vi "Calibrate xtal.vi"(5 "External Attenuation, dB":T8 format="%.2f", 7 "CART TCP Connection In":refnum<k5>, 8 "Error In":errorcluster, 9 "Max Input Power, dBm":T7 format="%.1f", 11 "RFSA Device":T16="RFSA") -> (0 "error out":errorcluster)   [LabVIEW 2011]
doc: "(c) Copyright 2006, National Instruments, Inc. This VI may not be duplicated, sold, or distributed without written consent from National Instruments."
uses:
  <userlib>/niRF/niSystem/SA/Includes/niSYS - RFSA - INC - STYP - Handle.ctl
  <userlib>/niRF/niSystem/SA/Includes/niSYS - SA - INC - STYP - Trigger.ctl
  <userlib>/niRF/niSystem/SA/Includes/niSYS - SA - INC - STYP - Trigger Delay.ctl
  <userlib>/niRF/niSystem/SA/Includes/niSYS - SA - INC - STYP - Timeout.ctl
  <userlib>/niRF/niBasic/SA/Spectrum/Includes/niBASIC - SA - Spectrum - INC - STYP - Averaging.ctl
  <userlib>/niRF/niBasic/SA/Spectrum/Includes/niBASIC - SA - Spectrum - INC - STYP - Measurement.ctl
  <userlib>/niRF/niSystem/SA/Includes/niSYS - SA - INC - STYP - Frequency Reference.ctl
  <userlib>/niRF/niSystem/SA/Includes/niSYS - SA - INC - STYP - External Attenuation.ctl
  <userlib>/niRF/niSystem/SA/Includes/niSYS - SA - INC - STYP - Max Input Power.ctl
  <userlib>/niRF/niSystem/SA/Includes/niSYS - SA - INC - STYP - Center Frequency.ctl
  <userlib>/niRF/niBasic/SA/Spectrum/Includes/niBASIC - SA - Spectrum - INC - STYP - FFT Window.ctl
  <userlib>/niRF/niBasic/SA/Spectrum/Includes/niBASIC - SA - Spectrum - INC - STYP - Measurement RBW.ctl
  <userlib>/niRF/niSystem/SA/Includes/niSYS - SA - INC - STYP - Span.ctl
  <userlib>/niRF/niBasic/SA/Spectrum/Includes/niBASIC - SA - Spectrum - INC - STYP - FFT Size.ctl
  <userlib>/niRF/niBasic/SA/Spectrum/Includes/niBASIC - SA - Spectrum - INC - STYP - Filter Type.ctl
  WLAN/UUT/QCA/Controls/QCA NART Response Type.ctl
  <userlib>/niRF/niBasic/SA/Spectrum/Includes/niBASIC - SA - Spectrum - INC - STYP - Measurement Trace Type.ctl
  <userlib>/niRF/niSystem/SA/Includes/niSYS - SA - INC - STYP - Measurement Request.ctl
panel:
  in  "Filter Type":T1
  in  "FFT Size":T2={"Auto"=enum."On", "Min Pnts/RBW"=3.1, "Window Length"=706, "FFT Length"=1024} {"Min Pnts/RBW" format="%.1f"}
  in  "Span, Hz":T3=1000000.0 format="%^.3e"
  in  "Measurement RBW, Hz":T4={"Auto"=enum."On", "RBW, Hz"=1000000.0} {"RBW, Hz" format="%^.3e"}
  in  "FFT Window":T5
  in  "RFSA Center Frequency, Hz":T6=2437000000.0 format="%^.6e"
  out "Spectrum Graph":T9(graph)={999501953.125, "Time Domain Interval, sec"=4882.8125, "Waveform Measurement Trace"=[-94.58885960127041, -96.86839023376476, -99.44994709212702, -95.73980201325817, -94.85468685558206, -93.89939819937095, -92.96907780368053, -94.62427677362473, -96.00114334271848, -95.0773520951145, -94.62079733063136, -95.66039665905808, -97.26831199401815, -94.4245843897965, -94.11636842862069, -93.58322383773326, -96.15404542236388, -96.24945397470107, -95.50507217914763, -96.54108841377801, -96.20009898290628, -94.5853296471187, -92.45746866418841, -91.28538347271048, -91.87185526400654, -94.56638317616594, -96.80701098668649, -98.3947929158942, -98.51183674015738, -97.19248581591714, -96.81596744977271, -95.42900485531823, -95.06526491233971, -94.58696887517611, -95.97070348701587, -96.12508871585825, -96.44070407370447, -95.79000716907146, -97.40271981045801, -96.56026806674593, -96.63105214105727, -95.37951512730523, -95.0709837906345, -97.57170348129546, -98.65428166191879, -92.85960027957853, -90.69744081914348, -91.78092902523147, -93.01528314210488, -94.00436029202501, -93.35100459361215, -93.65439480062977, -94.03853395069989, -94.46526514886557, -94.89042305851434, -94.67424970039717, -93.63794705250254, -92.45925730447641, -92.65908155014344, -93.60044471338867, -94.45278046002886, -94.14161306416081, -95.1968357622903, -94.78018101642988, -94.3521734655379, -93.66111421566106, -94.84863517357037, -94.5954023919716, -96.31573035476218, -96.10673186698642, -95.71535800929679, -94.23828099215436, -93.52563000159624, -95.57033866863337, -95.53015116793134, -93.56809331780974, -92.7606452725199, -93.57072573308072, -95.32780281550693, -92.86665354898099, -93.1370950166728, -94.12900193004297, -94.87833817452723, -94.72912032302605, -94.17479444496155, -94.72686892886344, -93.6596877329905, -92.66964149507194, -93.08938347771124, -94.20661112927449, -97.92818192608922, -94.73725815144995, -93.72795972831032, -95.83148845299667, -93.96304770180853, -93.50544784378508, -92.44166060977277, -93.27927003206689, -87.23502888503836, -72.11564523212036, -65.2815070033974, -63.751961771120435, -63.76202638288482, -64.94683436227825, -71.0137879230945, -85.10120059441533, -91.83446895184292, -90.61921828145796, -90.72235231920887, -91.03886336724534, -91.42747554368565, -91.50468859500515, -90.91036635524621, -91.23961076459484, -93.16256151029376, -95.66587614800164, -96.70895620214242, -94.44704301225457, -93.34996435212136, -92.18571998503167, -92.8876926563818, -93.5060742547249, -94.69941271506612, -97.92708620913864, -95.25428896670476, -92.62306680566677, -91.3874988202419, -91.85885903026352, -93.43215873965788, -94.90985702146794, -94.99607107512729, -94.53014477422813, -94.84999122998677, -95.93647533060847, -95.05672593509198, -97.64855424631322, -95.46215659926096, -94.67802340702697, -94.36305677166051, -95.093191185747, -95.15591730271399, -94.6393427453004, -95.01042716486224, -93.48932052409448, -93.1088259750116, -95.79379158863588, -94.27401403528606, -94.39185567902642, -95.78566610842289, -96.2278510846579, -97.35096719200405, -94.09028417116734, -93.67455962770373, -92.52661334344788, -92.28656403084389, -93.48717465263262, -95.87262940934153, -96.55075020577934, -96.23995801594376, -95.62432812173306, -95.53325913753295, -95.37316281463609, -96.84726282341614, -96.18759453809396, -92.65258606681302, -91.1549944641086, -91.18877556936353, -91.65922730189286, -92.7088197008887, -93.55252845804509, -93.23891521766758, -93.50579589024103, -93.22879114454076, -93.62878875149401, -94.89920966153908, -94.49841305989179, -94.31891446472981, -93.3315995436115, -92.9576487551588, -94.98762611566268, -97.76488288036198, -96.68686917193047, -95.69013350308543, -95.23811265655995, -95.43343805014592, -96.1176286234256, -98.40428345012647, -97.1939542411557, -93.8709557440311, -92.5732899687502, -93.19402090455232, -93.4806645014271, -92.62376136260087, -93.4169081651324, -95.1135305356191, -95.44327303741449, -95.97664612099189, -95.20918978347628, -93.30477056749844, -92.75514488033883, -92.92596032798458, -94.3147334729053, -95.75765916034278, -97.49920812243585, -93.12822887068018]}
  in  "Frequency Reference":T10={" Reference Source"=enum."On Board Clock", "Frequency, Hz"=10000000.0, "Backplane Source"=enum."None"} {"Frequency, Hz" format="%^.6e"}
  out "Spectrum Measurement":T11={"Peak Amplitude, dBm"=-63.751961771120435, "Peak Frequency, Hz"=999995117.1875, "Number of Points"=256, "Start Frequency, Hz"=999501953.125, "Space Frequency, Hz"=4882.8125} {"Space Frequency, Hz" format="%^.6e"; "Start Frequency, Hz" format="%^.6e"; "Peak Frequency, Hz" format="%^.6e"; "Peak Amplitude, dBm" format="%.2f"}
  in  "Spectrum Averaging":T12={"Averages"=10, "Average State"=enum."On", "Average Mode"=enum."Repeat", "Average Type"=enum."Log"}
  in  "Timeout, sec":T13=10.0 format="%.3f"
  in  "Trigger":T14={"Source"=enum."Immediate", "Edge"=enum."Rising", "Delay, sec"=0.0, "Level, dBm"=-20.0, "Min Quiet Time, sec"=0.0} {"Min Quiet Time, sec" format="%^.2e"; "Level, dBm" format="%.1f"; "Delay, sec" format="%^.2e"}
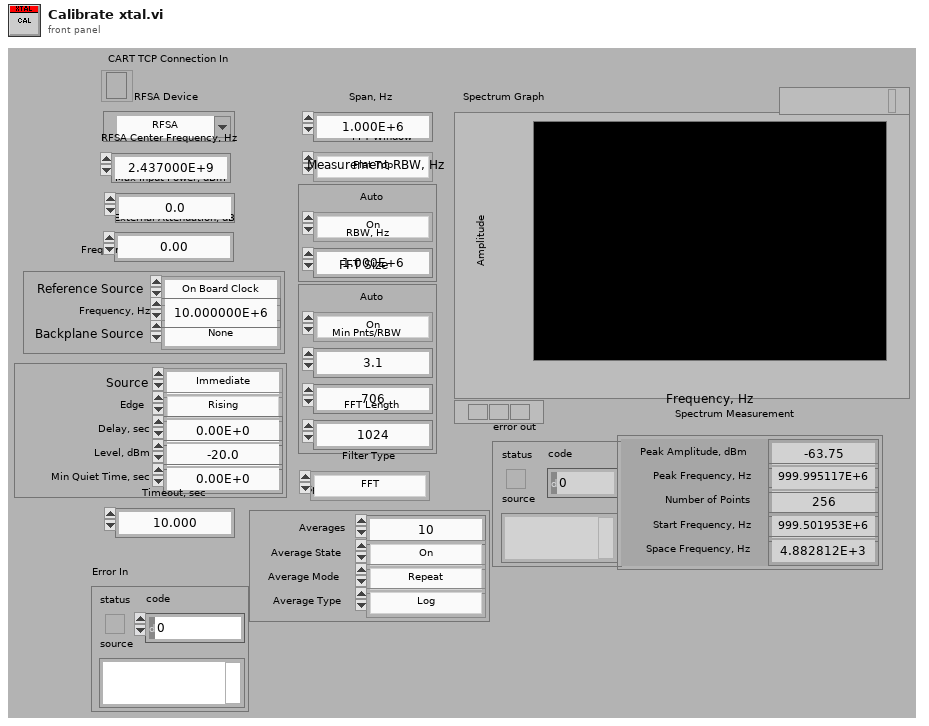
[diagram p1: front panel]
types:
  T1 = typedef "niBASIC - SA - Spectrum - INC - STYP - Filter Type.ctl" = enum16{"FFT", "5-Pole", "Gaussian"}
  T2 = typedef "niBASIC - SA - Spectrum - INC - STYP - FFT Size.ctl" = cluster{"Auto":enum16{"Off", "On"}, "Min Pnts/RBW":dbl, "Window Length":i32, "FFT Length":i32}
  T3 = typedef "niSYS - SA - INC - STYP - Span.ctl" = dbl
  T4 = typedef "niBASIC - SA - Spectrum - INC - STYP - Measurement RBW.ctl" = cluster{"Auto":enum16{"Off", "On"}, "RBW, Hz":dbl}
  T5 = typedef "niBASIC - SA - Spectrum - INC - STYP - FFT Window.ctl" = enum16{"Flat Top", "Uniform", "Hanning", "Hamming", "Gaussian", "Blackman", "Blackman-Harris", "Kaiser-Bessel 70 dB", "Kaiser-Bessel 90 dB", "Kaiser-Bessel 110 dB"}
  T6 = typedef "niSYS - SA - INC - STYP - Center Frequency.ctl" = dbl
  T7 = typedef "niSYS - SA - INC - STYP - Max Input Power.ctl" = dbl
  T8 = typedef "niSYS - SA - INC - STYP - External Attenuation.ctl" = dbl
  T9 = cluster{dbl, "Time Domain Interval, sec":dbl, "Waveform Measurement Trace":dbl[]}
  T10 = typedef "niSYS - SA - INC - STYP - Frequency Reference.ctl" = cluster{" Reference Source":enum16{"On Board Clock", "Ref In", "PXI Clock 10"}, "Frequency, Hz":dbl, "Backplane Source":enum16{"None", "Ref In", "On Board Clock"}}
  T11 = typedef "niBASIC - SA - Spectrum - INC - STYP - Measurement.ctl" = cluster{"Peak Amplitude, dBm":dbl, "Peak Frequency, Hz":dbl, "Number of Points":i32, "Start Frequency, Hz":dbl, "Space Frequency, Hz":dbl}
  T12 = typedef "niBASIC - SA - Spectrum - INC - STYP - Averaging.ctl" = cluster{"Averages":i32, "Average State":enum16{"Off", "On"}, "Average Mode":enum16{"Exponential", "Repeat"}, "Average Type":enum16{"RMS", "Log", "Scalar", "Max", "Min"}}
  T13 = typedef "niSYS - SA - INC - STYP - Timeout.ctl" = dbl
  T14 = typedef "niSYS - SA - INC - STYP - Trigger.ctl" = cluster{"Source":enum16{"Immediate", "External", "Software", "RTSI 0", "RTSI 1", "RTSI 2", "RTSI 3", "RTSI 4", "RTSI 5", "RTSI 6", "RTSI 7", "PFI 0", "PFI 1", "PFI 2", "PXI Star", "Power"}, "Edge":enum16{"Rising", "Falling"}, "Delay, sec":T15, "Level, dBm":dbl, "Min Quiet Time, sec":dbl}
  T15 = typedef "niSYS - SA - INC - STYP - Trigger Delay.ctl" = dbl
  T16 = typedef "niSYS - RFSA - INC - STYP - Handle.ctl" = refnum<k15>
  T17 = typedef "niBASIC - SA - Spectrum - INC - STYP - Measurement Handle.ctl" = refnum<notifier>
  T18 = typedef "QCA NART Response Type.ctl" = enum16{"DEBUG", "CONTROL", "INFO", "WARNING", "ERROR", "NONE"}
  T19 = typedef "niBASIC - SA - Spectrum - INC - STYP - Measurement Trace Type.ctl" = enum16{"Unprocessed I/Q", "Measurements", "Average Spectrum"}
  T20 = typedef "niSYS - SA - INC - STYP - Measurement Request.ctl" = enum16{"Measure", "Fetch", "Initiate"}
  T21 = typedef "niSYS - SA - INC - STYP - Measurement Trace.ctl" = dbl[]
  T22 = typedef "niSYS - SA - INC - STYP - Real Waveform.ctl" = cluster{"x0":dbl, "dx":dbl, "y":dbl[]}
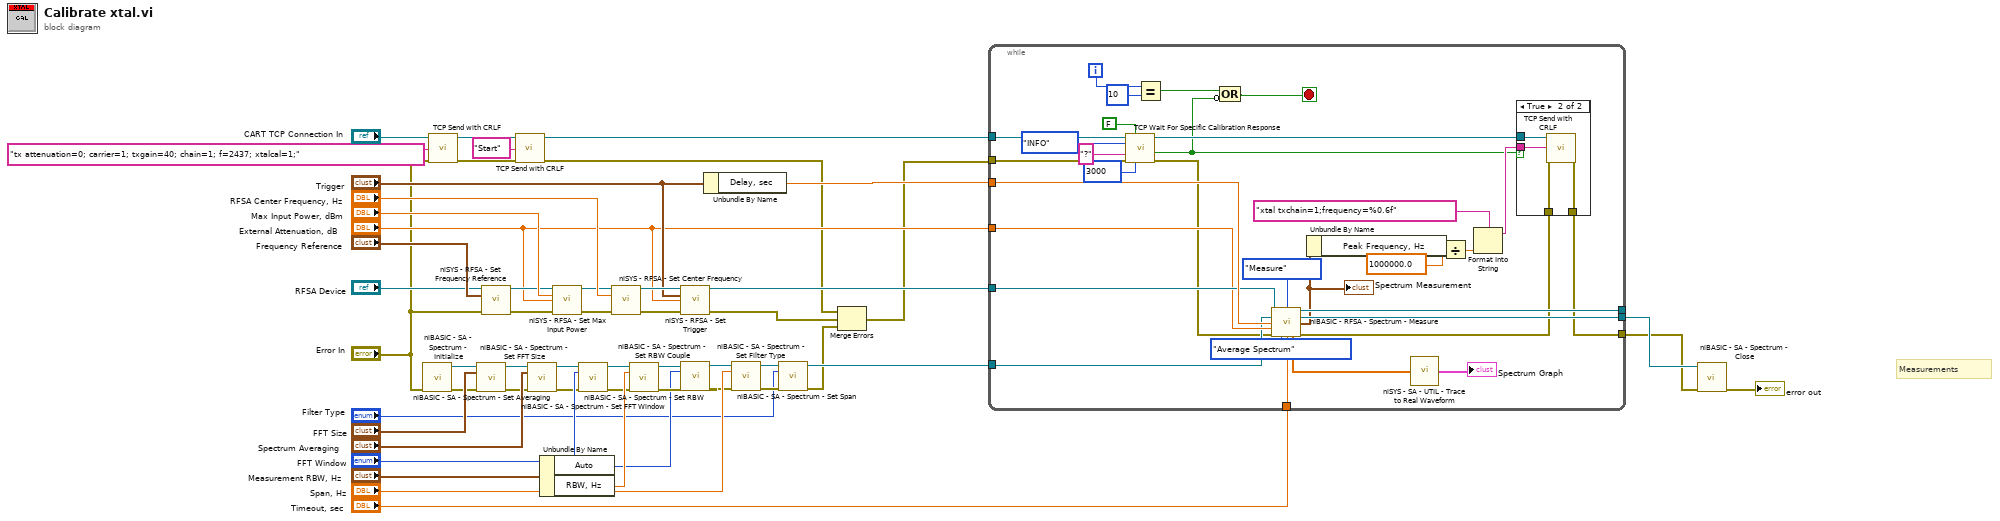
[diagram p0: block diagram]
diagram:
  # "Measurements"
  n1 = call <userlib>:"niBASIC - SA - Spectrum - Initialize.vi"("error in (no error)"="Error In") -> ("Measurement Handle Out"=w27:T17, "error out"=w28:errorcluster)  [unwired: 1 in, 12 out]
  n2 = call "TCP Send with CRLF.vi"("CART TCP Connection"="CART TCP Connection In", "data in"="tx attenuation=0; carrier=1; txgain=40; chain=1; f=2437; xtalcal=1;", "error IO"="Error In") -> ("CART TCP Connection Out"=w8:refnum<k5>, "error out"=w9:errorcluster)  [unwired: 11 in]
  n3 = call <userlib>:"niBASIC - SA - Spectrum - Set FFT Size.vi"("Measurement Handle In"=w27, "FFT Size"="FFT Size", "error in (no error)"=w28) -> ("Measurement Handle Out"=w41:T17, "error out"=w42:errorcluster)  [unwired: 11 out]
  n4 = call <userlib>:"niSYS - RFSA - Set Frequency Reference.vi"("RFSA Handle In"="RFSA Device", "Frequency Reference"="Frequency Reference", "error in (no error)"="Error In") -> ("RFSA Handle Out"=w30:T16, "error out"=w29:errorcluster)  [unwired: 1 in, 10 out]
  n5 = call "TCP Send with CRLF.vi"("CART TCP Connection"=w8, "data in"="Start", "error IO"=w9) -> ("CART TCP Connection Out"=w6:refnum<k5>, "error out"=w5:errorcluster)  [unwired: 11 in]
  n6 = call <userlib>:"niBASIC - SA - Spectrum - Set Averaging.vi"("Measurement Handle In"=w41, "Averaging"="Spectrum Averaging", "error in (no error)"=w42) -> ("Measurement Handle Out"=w39:T17, "error out"=w40:errorcluster)  [unwired: 11 out]
  n7 = Unbundle By Name("Measurement RBW, Hz") -> ("Auto"=w31:enum16{"Off", "On"}, "RBW, Hz"=w38:dbl)
  n8 = call <userlib>:"niSYS - RFSA - Set Max Input Power.vi"("RFSA Handle In"=w30, "Max Input Power, dBm"="Max Input Power, dBm", "External Attenuation, dB"="External Attenuation, dB", "error in (no error)"=w29) -> ("RFSA Handle Out"=w43:T16, "error out"=w44:errorcluster)  [unwired: 10 out]
  n9 = call <userlib>:"niBASIC - SA - Spectrum - Set FFT Window.vi"("Measurement Handle In"=w39, "FFT Window"="FFT Window", "error in (no error)"=w40) -> ("Measurement Handle Out"=w36:T17, "error out"=w37:errorcluster)  [unwired: 11 out]
  n10 = call <userlib>:"niSYS - RFSA - Set Center Frequency.vi"("RFSA Handle In"=w43, "RFSA Center Frequency, Hz"="RFSA Center Frequency, Hz", "error in (no error)"=w44) -> ("RFSA Handle Out"=w25:T16, "error out"=w26:errorcluster)  [unwired: 11 out]
  n11 = call <userlib>:"niBASIC - SA - Spectrum - Set RBW.vi"("Measurement Handle In"=w36, "RBW, Hz"=w38, "error in (no error)"=w37) -> ("Measurement Handle Out"=w33:T17, "error out"=w35:errorcluster)  [unwired: 11 out]
  n12 = call <userlib>:"niSYS - RFSA - Set Trigger.vi"("RFSA Handle In"=w25, "Trigger"="Trigger", "External Attenuation, dB"="External Attenuation, dB", "error in (no error)"=w26) -> ("RFSA Handle Out"=w22:T16, "error out"=w17:errorcluster)  [unwired: 10 out]
  n13 = call <userlib>:"niBASIC - SA - Spectrum - Set RBW Couple.vi"("Measurement Handle In"=w33, "Auto"=w31, "error in (no error)"=w35) -> ("Measurement Handle Out"=w32:T17, "error out"=w34:errorcluster)  [unwired: 11 out]
  n14 = Unbundle By Name("Trigger") -> ("Delay, sec"=w23:T15)
  n15 = call <userlib>:"niBASIC - SA - Spectrum - Set Span.vi"("Measurement Handle In"=w32, "Span, Hz"="Span, Hz", "error in (no error)"=w34) -> ("Measurement Handle Out"=w16:T17, "error out"=w14:errorcluster)  [unwired: 11 out]
  n16 = call <userlib>:"niBASIC - SA - Spectrum - Set Filter Type.vi"("Measurement Handle In"=w16, "Filter Type"="Filter Type", "error in (no error)"=w14) -> ("Measurement Handle Out"=w15:T17, "error out"=w13:errorcluster)  [unwired: 10 in, 1 out]
  n17 = Merge Errors(w5, w17, w13) -> (w4:errorcluster)
  n18 = while {
    tunnel: w23 -> [w84]
    tunnel: w22 -> [w83]
    tunnel: "External Attenuation, dB" -> [w82]
    tunnel: "Timeout, sec" -> [w79]
    tunnel: [w78] -> _
    tunnel: [w55] -> w1
    tunnel: [w77] -> w19
    tunnel: w15 -> [w76]
    tunnel: w6 -> [w65]
    tunnel: w4 -> [w64]
    i -> [w61]
    stop <- w57 stop-if-true
    n19 = call "TCP Wait For Specific Calibration Response.vi"("TCP Connection In"=w65, "Next response (t)"=FALSE, "Expected Type"=QCA_NART_Response_Type."INFO", "Expected Message Start (\"\":any)"="?" ("Expected Message Start (\"\":any)"), "error in"=w64, "Timeout (250 ms)"=3000) -> ("TCP Connection Out"=w66:refnum<k5>, "More Pwr Reporting?"=w59:bool, "error out"=w62:errorcluster)  [unwired: 5 in, 2 out]
    n20 = Equal?(x=w61, y=10) -> (x = y?=w58:bool)
    n21 = Compound Arithmetic op=OR(w58, invert w59) -> (w57:bool)
    n22 = call <userlib>:"niBASIC - RFSA - Spectrum - Measure.vi"("RFSA Handle In"=w83, "Measurement Request"=niSYS_-_SA_-_INC_-_STYP_-_Measurement_Request."Measure", "Measurement Handle In"=w76, "Trigger Delay, sec"=w84, "External Attenuation, dB"=w82, "error in (no error)"=w62, "Measurement Trace Type"=niBASIC_-_SA_-_Spectrum_-_INC_-_STYP_-_Measurement_Trace_Type."Average Spectrum", "Timeout, sec"=w79) -> ("RFSA Handle Out"=w78:T16, "Measurement Handle Out"=w77:T17, "Measurement"=w75:T11, "Measurement Trace"=w53:T21, "error out"=w56:errorcluster)  [unwired: 3 out]
    "Spectrum Measurement" <- w75
    n23 = Unbundle By Name(w75) -> ("Peak Frequency, Hz"=w72:dbl)
    n24 = call <userlib>:"niSYS - SA - UTIL - Trace to Real Waveform.vi"("Measurement Trace"=w53) -> ("Signal"=→"Spectrum Graph":T22)
    n25 = Divide(x=w72, y=1000000.0) -> (x/y=w71:dbl)
    n26 = Format Into String(format string="xtal txchain=1;frequency=%0.6f", w71) -> (resulting string=w73:string)  [unwired: 2 in, 1 out]
    n27 = case shown="True" w59 {
      tunnel: w66 -> [_ w89]
      tunnel: w73 -> [_ w88]
      tunnel: w56 -> [w85 w87]
      tunnel: [w85 w86] -> w55
      frame False {
      }
      frame True {
        n28 = call "TCP Send with CRLF.vi"("CART TCP Connection"=w89, "data in"=w88, "error IO"=w87) -> ("error out"=w86:errorcluster)  [unwired: 11 in, 1 out]
      }
    }
  }
  n29 = call <userlib>:"niBASIC - SA - Spectrum - Close.vi"("Measurement Handle In"=w19, "error in (no error)"=w1) -> ("error out"=→"error out":errorcluster)  [unwired: 13 out]
